vi "Dummy Error Cluster from Error Code.vi"(8 "error in (no error)":errorcluster, 10 "Boolean":bool, 11 "Actor in":refnum<class "Actor.lvclass">) -> (0 "error out":errorcluster, 5 "Boolean 3":bool, 7 "Boolean 2":bool)   [LabVIEW 2016]
uses:
  <vilib>/ActorFramework/Actor/Actor.lvclass
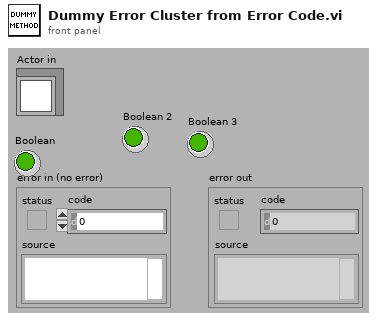
[diagram p1: front panel]
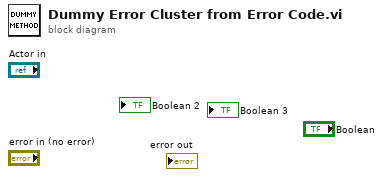
[diagram p0: block diagram]
diagram:
